vi "dscADSampleAvg.vi"(8 "error in":errorcluster, 10 "count":i32, 11 "board":i16) -> (0 "error out":errorcluster, 1 "Avg":dbl, 2 "numAvg":i32, 3 "boardOut":i16)   [LabVIEW 2011, in "Diamond Universal Driver.lvlib"]
doc: "Perform fixed number (defined by <B>count</B>) of A/D conversions on the currently selected channel and return the average. The function first waits for the board to be ready for a conversion, then starts the conversion and wiats for it to finish before reading the data from the board. A built-in timer is used to check the for board failure. If the timer times out before the conversion completes, the board returns the error code."
uses:
  Diamond Universal Driver.lvlib
  Controls/error codes.ctl
  Instruments/WL OPC/Support/dlls/dscud.dll
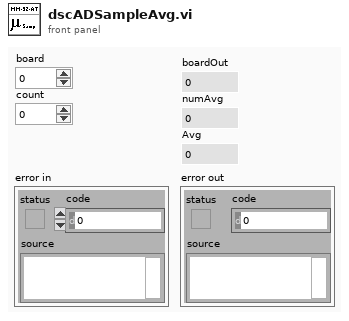
[diagram p1: front panel]
types:
  T1 = typedef "Diamond Universal Driver.lvlib/error codes.ctl" = enum8{"DE_NONE", "DE_HW_FAILURE", "DE_SW_FAILURE", "DE_HW_NOT_SUPPORTED", "DE_SW_NOT_SUPPORTED", "DE_INVALID_PARM", "DE_ALTERNATE_IN_PROGRESS", "DE_NONE_IN_PROGRESS", "DE_BUFFER_ROLLOVER", "DE_INVALID_ERROR_CODE", "DE_ALREADY_PAUSED", "DE_OVERFLOW", "DE_INVALID_FUNC", "DE_DSCUDH_INVALID", "DE_INVALID_BOARD", "DE_BOARD_LIMIT_REACHED", "DE_BOARD_BUSY", "DE_INVALID_WINDRVR_HANDLE", "DE_INVALID_WINDRVR_VERSION", "DE_BAD_WINDRVR_BOARD_INIT", "DE_OPERATION_TIMED_OUT", "DE_INVALID_WINDRVR_KP", "DE_THREAD_FAILURE"}
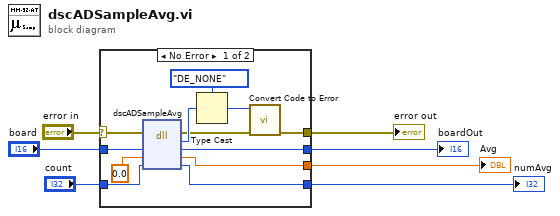
[diagram p0: block diagram]
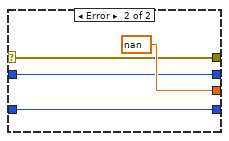
[diagram p2: hidden frame]
diagram:
  n1 = case shown="No Error" "error in" {
    selector: "error in" -> [w19 w20]
    tunnel: "count" -> [w18 w23]
    tunnel: "board" -> [w17 w21]
    tunnel: [w16 nan] -> w4
    tunnel: [w15 w21] -> w3
    tunnel: [w14 w23] -> w2
    tunnel: [w9 w20] -> w1
    frame No Error {
      n2 = dll-call lib="C:/Users/mrichardson/Documents/Web Based Version Control SW/Instruments/WL OPC/Support/dlls/dscud.dll" fn="dscADSampleAvg"(error in=w19, "board"=w17, 0.0, "count"=w18) -> (error out=w11:errorcluster, "error"=w13:u8, "board"=w15:i16, w16:dbl, "count"=w14:i32)  [unwired: 2 in, 1 out]
      n3 = Type Cast(type=error_codes."DE_NONE" ("error codes"), x=w13) -> (*(type *) &x=w10:T1)
      n4 = call "Convert Code to Error.vi"("error in"=w11, "error codes"=w10) -> ("error out"=w9:errorcluster)  [unwired: 9 in]
    }
    frame Error {
    }
  }
  "boardOut" <- w3
  "numAvg" <- w2
  "Avg" <- w4
  "error out" <- w1
